vi "GenerateID.vi"() -> (3 "id":i32)   [LabVIEW 2013, in "SMO.jsonRPC.lvclass"]
uses:
  SMO.jsonRPC.lvclass
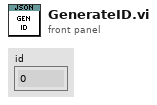
[diagram p1: front panel]
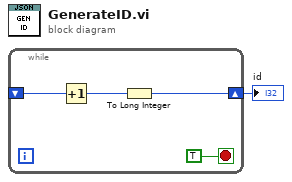
[diagram p0: block diagram]
diagram:
  n1 = while {
    shift-right: [w3] -> w1
    shift-left: _ -> [w5]
    stop <- TRUE stop-if-true
    n2 = Increment(x=w5) -> (x+1=w4:i32)
    n3 = To Long Integer(number=w4) -> (32bit integer=w3:i32)
  }
  "id" <- w1
